vi "InitHisto.vi"(6 "lencode":i32, 7 "tacq":i32, 8 "error in (no error)":errorcluster, 9 "Offset":i32, 10 "Binning":i32 min=0 max=8 step=1, 11 "Multiharp in":refnum<class "Multiharp.lvclass">) -> (0 "error out":errorcluster, 3 "Multiharp out":refnum<class "Multiharp.lvclass">)   [LabVIEW 2023, in "Multiharp.lvlib" / "Multiharp.lvclass"]
uses:
  Multiharp.lvclass
  MultiharpComm Messages/MH_ChannelInitDone Msg/MH_ChannelInitDone Msg.lvclass
  <vilib>/ActorFramework/Actor/Actor.lvclass
panel:
  in  "event data 2":cluster{"Init":bool, "nchannels":i32}
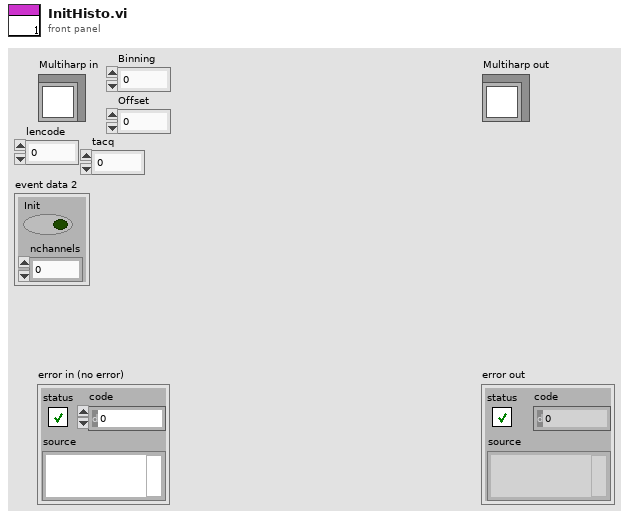
[diagram p1: front panel]
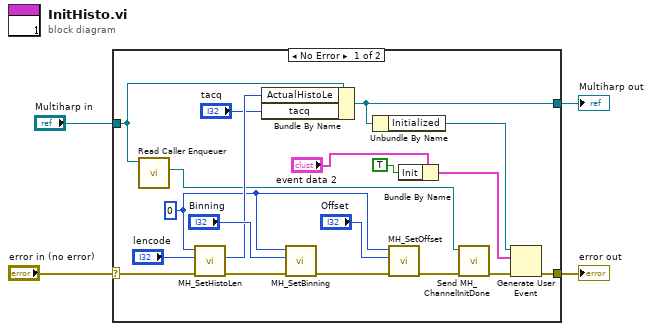
[diagram p0: block diagram]
diagram:
  n1 = case shown="No Error" "error in (no error)" {
    selector: "error in (no error)" -> [w18 w24]
    tunnel: [w5 w25] -> w2
    tunnel: "Multiharp in" -> [w8 w25]
    tunnel: [w6 w24] -> w1
    frame No Error {
      w16 = 0 ("devidx")
      n2 = call <vilib>:"Read Caller Enqueuer.vi"("Actor"=w8) -> ("Caller Enqueuer"=w15:refnum<class "Message Enqueuer.lvclass">)  [unwired: 10 in]
      n3 = call "MH_SetHistoLen.vi"("error in (no error)"=w18, "lencode"="lencode", "devidx"=w16) -> ("error out"=w19:errorcluster, "actuallen"=w17:i32)  [unwired: 6 in, 1 out]
      n4 = Bundle By Name(cluster=w8, "ActualHistoLe"=w17, "tacq"="tacq") -> (w5:refnum<class "Multiharp.lvclass">)
      n5 = call "MH_SetBinning.vi"("error in (no error)"=w19, "Binning"="Binning", "devidx"=w16) -> ("error out"=w20:errorcluster)  [unwired: 7 in, 1 out]
      n6 = Unbundle By Name(w5) -> ("Initialized"=w10:refnum<user-event>)
      n7 = call "MH_SetOffset.vi"("error in (no error)"=w20, "Offset"="Offset", "devidx"=w16) -> ("error out"=w14:errorcluster)  [unwired: 7 in, 1 out]
      n8 = Bundle By Name(cluster="event data 2", "Init"=TRUE) -> (w11:cluster{"Init":bool, "nchannels":i32})
      n9 = call "Send MH_ChannelInitDone.vi"("error in (no error)"=w14, "Message Enqueuer"=w15) -> ("error out"=w7:errorcluster)  [unwired: 8 in, 1 out]
      n10 = Generate User Event(user event=w10, event data cluster=w11, error in=w7) -> (error out=w6:errorcluster)  [unwired: 1 in, 1 out]
    }
    frame Error {
    }
  }
  "error out" <- w1
  "Multiharp out" <- w2
